vi "Kinesis-program-one-motor.vi"() -> ()   [LabVIEW 2014]
doc: "André Romero - 2017\nandretec@ifsc.usp.br"
panel:
  out "Line (mm/s)":dbl
  out "GetPOS":dbl format="%#_6f"
  out "Numeric":i32
  out "IsMoving":bool
  out "GetPOS X":dbl=10.0 format="%^#1_6e"
  in  "GO Move":bool
  out "Motor 1":bool
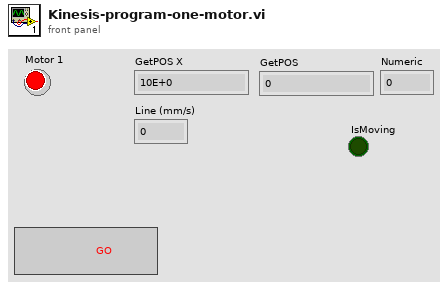
[diagram p1: front panel]
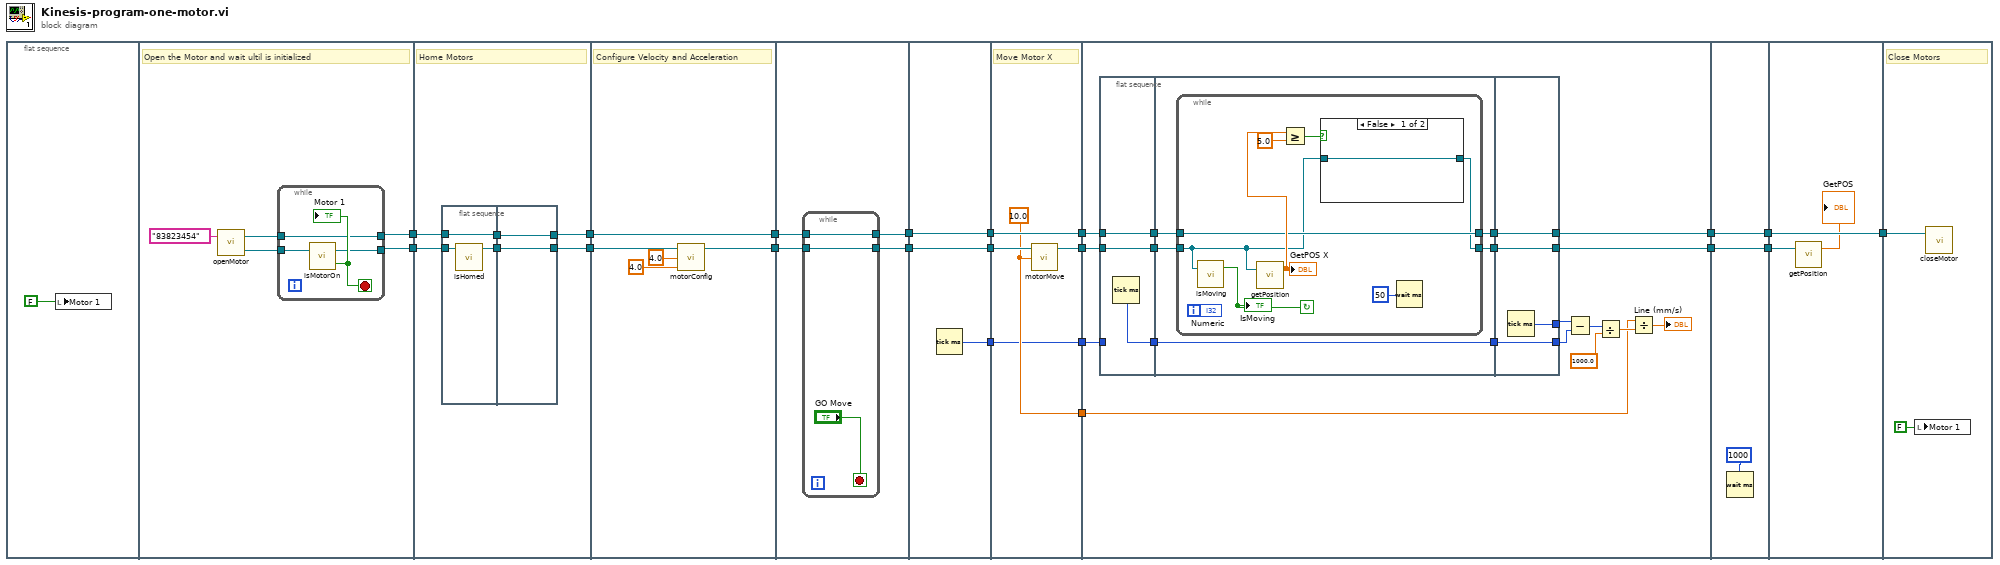
[diagram p0: block diagram]
diagram:
  n1 = flat-sequence {
    tunnel: [w26] -> w9
    tunnel: [w25] -> w8
    tunnel: w9 -> [w36]
    tunnel: w8 -> [w35]
    tunnel: [w33] -> w20
    tunnel: [w32] -> w18
    tunnel: w20 -> [w46]
    tunnel: [w46] -> w19
    tunnel: w18 -> [w42]
    tunnel: [w43] -> w17
    tunnel: w19 -> [w50]
    tunnel: [w49] -> w4
    tunnel: w17 -> [w47]
    tunnel: [w48] -> w6
    tunnel: w6 -> [w56]
    tunnel: [w56] -> w5
    tunnel: w4 -> [w55]
    tunnel: [w55] -> w3
    tunnel: [w54] -> w1
    tunnel: w5 -> [w60]
    tunnel: [w59] -> w16
    tunnel: w3 -> [w61]
    tunnel: [w61] -> w15
    tunnel: [w58] -> w7
    tunnel: [w57] -> w2
    tunnel: w1 -> [w57]
    tunnel: w16 -> [w76]
    tunnel: [w77] -> w14
    tunnel: w15 -> [w79]
    tunnel: [w78] -> w13
    tunnel: w7 -> [w64]
    tunnel: w2 -> [w62]
    tunnel: w14 -> [w105]
    tunnel: [w105] -> w12
    tunnel: w13 -> [w104]
    tunnel: [w104] -> w11
    tunnel: w12 -> [w107]
    tunnel: w11 -> [w108]
    tunnel: [w108] -> w10
    tunnel: w10 -> [w110]
    frame #0 {
      n2 = local write "Motor 1"(FALSE ("isConnected")) -> ()
    }
    frame #1 {
      # "Open the Motor and wait ultil is initialized"
      n3 = call "openMotor.vi"("S/N Motor"="83823454") -> ("Device"=w23:refnum<k24>, ".NET Refnum out"=w24:refnum<k24>)  [unwired: 1 in]
      n4 = while {
        tunnel: [w29] -> w26
        tunnel: [w27] -> w25
        tunnel: w24 -> [w29]
        tunnel: w23 -> [w28]
        stop <- w30 stop-if-true
        n5 = call "isMotorOn.vi"("Device"=w28) -> ("isConnected"=w30:bool, "Device out"=w27:refnum<k24>)  [unwired: 1 in]
        "Motor 1" <- w30
      }
    }
    frame #2 {
      # "Home Motors"
      n6 = flat-sequence {
        tunnel: w36 -> [w39]
        tunnel: w35 -> [w38]
        tunnel: [w39] -> w34
        tunnel: [w37] -> w31
        tunnel: [w40] -> w32
        tunnel: [w41] -> w33
        tunnel: w34 -> [w41]
        tunnel: w31 -> [w40]
        frame #0 {
          n7 = call "isHomed.vi"("Device in"=w38) -> ("Device out"=w37:refnum<k24>)  [unwired: 4 in]
        }
        frame #1 {
        }
      }
    }
    frame #3 {
      # "Configure Velocity and Acceleration"
      n8 = call "motorConfig.vi"("Velocity"=4.0 ("MaxVelocity"), "Acceleration"=4.0, "Device in"=w42) -> ("Device out"=w43:refnum<k24>)  [unwired: 2 in]
    }
    frame #4 {
      n9 = while {
        tunnel: [w52] -> w49
        tunnel: w50 -> [w52]
        tunnel: [w51] -> w48
        tunnel: w47 -> [w51]
        stop <- "GO Move" stop-if-true
      }
    }
    frame #5 {
      n10 = Tick Count (ms)() -> (millisecond timer value=w54:u32)
    }
    frame #6 {
      w58 = 10.0 ("position")
      # "Move Motor X"
      n11 = call "motorMove.vi"("position"=w58, "Device in"=w60) -> ("Device out"=w59:refnum<k24>)  [unwired: 3 in]
    }
    frame #7 {
      n12 = flat-sequence {
        tunnel: w76 -> [w81]
        tunnel: w79 -> [w82]
        tunnel: [w82] -> w75
        tunnel: [w81] -> w74
        tunnel: [w80] -> w68
        tunnel: w62 -> [_]
        tunnel: w75 -> [w87]
        tunnel: w74 -> [w84]
        tunnel: [w86] -> w73
        tunnel: [w85] -> w72
        tunnel: [w83] -> w69
        tunnel: w68 -> [w83]
        tunnel: [w101] -> w77
        tunnel: [w102] -> w78
        tunnel: w73 -> [w102]
        tunnel: w72 -> [w101]
        tunnel: [w100] -> w71
        tunnel: [w99] -> w70
        tunnel: w69 -> [w99]
        frame #0 {
          n13 = Tick Count (ms)() -> (millisecond timer value=w80:u32)
        }
        frame #1 {
          n14 = while {
            tunnel: w87 -> [w90]
            tunnel: w84 -> [w89]
            tunnel: [w90] -> w86
            tunnel: [w88] -> w85
            i -> [w95]
            stop <- w96 continue-if-true
            n15 = call "isMoving.vi"("Device in"=w89) -> ("IsMoving"=w96:bool)  [unwired: 1 in, 1 out]
            "IsMoving" <- w96
            n16 = call "getPosition.vi"("Device"=w89) -> ("GetPOS"=w93:dbl)  [unwired: 2 in]
            "GetPOS X" <- w93
            n17 = Greater Or Equal?(x=w93, y=5.0) -> (x >= y?=w91:bool)
            n18 = case shown="False" w91 {
              tunnel: w89 -> [w97 w98]
              tunnel: [w97 w98] -> w88
              frame False {
              }
              frame True {
              }
            }
            n19 = Wait (ms)(milliseconds to wait=u32 50) -> ()  [unwired: 1 out]
            "Numeric" <- w95
          }
        }
        frame #2 {
          n20 = Tick Count (ms)() -> (millisecond timer value=w100:u32)
        }
      }
      n21 = Subtract(x=w71, y=w70) -> (x-y=w67:u32)
      n22 = Divide(x=w67, y=1000.0) -> (x/y=w65:dbl)
      n23 = Divide(x=w64, y=w65) -> (x/y=→"Line (mm/s)":dbl)
    }
    frame #8 {
      n24 = Wait (ms)(milliseconds to wait=u32 1000) -> ()  [unwired: 1 out]
    }
    frame #9 {
      n25 = call "getPosition.vi"("Device"=w107) -> ("GetPOS"=→"GetPOS":dbl)  [unwired: 2 in]
    }
    frame #10 {
      # "Close Motors"
      n26 = local write "Motor 1"(FALSE ("Motor 1")) -> ()
      n27 = call "closeMotor.vi"(".NET Refnum in"=w110) -> ()  [unwired: 2 in]
    }
  }
